vi "Create Transfer Group.vi"(4 "engine offset":u64, 5 "Debug Flags":refnum<class "Debug Flags.lvclass">, 6 "transceiver id":i32, 7 "framework id":i32, 8 "error in (no error)":errorcluster, 9 "Direction":T1, 10 "Timing":refnum<class "Engine Timing.lvclass">, 11 "Transfers":refnum<class "Transfer.lvclass">[](array[class])) -> (0 "error out":errorcluster, 3 "Transfer Group out":refnum<class "Transfer Group.lvclass">)   [LabVIEW 2017, in "Data Sharing Framework Core.lvlib" / "Data Sharing Framework Engine.lvlib" / "Transfer Group.lvclass"]
uses:
  Transfer Group.lvclass
  Transfer/Transfer.lvclass
  Internal/Timing/Engine Timing.lvclass
  Configuration/1.0.0/Public/Controls/DSF Direction.ctl
  Internal/Debug/Debug Flags/Debug Flags.lvclass
  Transfer Group.lvclass/Transfer Group.ctl
  Configuration/1.0.0/Data Sharing Framework Configuration.lvlib
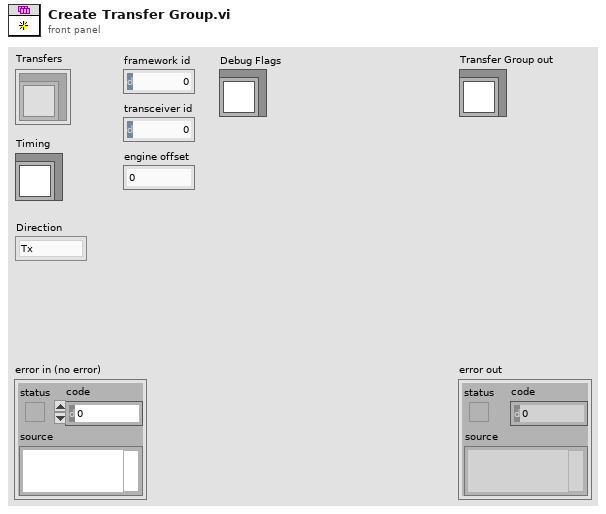
[diagram p1: front panel]
types:
  T1 = typedef "Data Sharing Framework Core.lvlib/Data Sharing Framework Configuration.lvlib/DSF Direction.ctl" = enum8{"Tx", "Rx"}
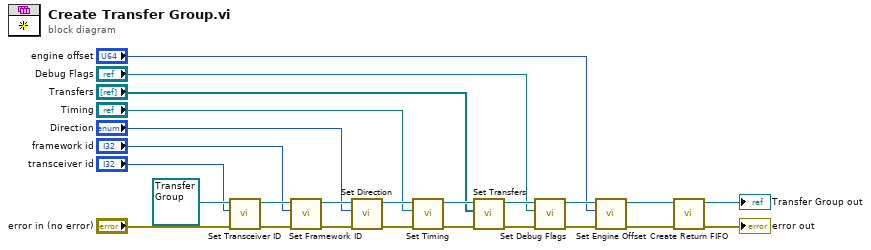
[diagram p0: block diagram]
diagram:
  n1 = call "Set Transceiver ID.vi"("transceiver id"="transceiver id", "Transfer Group in"=refnum<class "Transfer Group.lvclass"> refnum ("Transfer Group type")) -> ("Transfer Group out"=w7:refnum<class "Transfer Group.lvclass">)  [unwired: 9 in]
  n2 = call "Set Framework ID.vi"("framework id"="framework id", "Transfer Group in"=w7) -> ("Transfer Group out"=w18:refnum<class "Transfer Group.lvclass">)  [unwired: 9 in]
  n3 = call "Set Direction.vi"("Direction"="Direction", "Transfer Group in"=w18) -> ("Transfer Group out"=w17:refnum<class "Transfer Group.lvclass">)  [unwired: 9 in]
  n4 = call "Set Timing.vi"("Timing"="Timing", "Transfer Group in"=w17) -> ("Transfer Group out"=w16:refnum<class "Transfer Group.lvclass">)  [unwired: 9 in]
  n5 = call "Set Transfers.vi"("Transfers"="Transfers", "Transfer Group in"=w16) -> ("Transfer Group out"=w9:refnum<class "Transfer Group.lvclass">)  [unwired: 9 in]
  n6 = call "Set Debug Flags.vi"("Debug Flags"="Debug Flags", "Transfer Group in"=w9) -> ("Transfer Group out"=w3:refnum<class "Transfer Group.lvclass">)  [unwired: 9 in]
  n7 = call "Set Engine Offset.vi"("engine offset"="engine offset", "Transfer Group in"=w3) -> ("Transfer Group out"=w2:refnum<class "Transfer Group.lvclass">)  [unwired: 9 in]
  n8 = call "Create Return FIFO.vi"("error in (no error)"="error in (no error)", "Transfer Group in"=w2) -> ("error out"=→"error out":errorcluster, "Transfer Group out"=→"Transfer Group out":refnum<class "Transfer Group.lvclass">)  [unwired: 8 in]
